vi "prep cmrcial shots report (SubVI).vi"(0 "reportType":enum32{"V50", "NIJ"}(ring), 1 "language":enum16{"Spanish", "Portuguese", "English"}(ring), 2 "shotsArr":T1 {"Frag Rod" format="%.1f"; "UncorrectedAvgVel_PB" format="%.1f"; "UncorrectedRed_PB" format="%.1f"; "strikeVel_PB" format="%.1f"; "velLoss_PB" format="%.1f"; "avgVel_PB" format="%.1f"; "Redundant_Velocity" format="%.1f"; "Energy Loss (J)" format="%.3e"; "Projectile Mass" min=0 step=1 format="%.4f"; "Corrected residual" format="%.2f"; "Uncorrected Residual" format="%.1f"; "Corrected Impact" format="%.2f"; "Uncorrected Impact" format="%.1f"; "Shot Angle" max=90 step=1; "SHOT STATUS" items=["Partial", "Complete"]; "IMPACT VELOCITY" min=0 max=10000 step=0.1 format="%.1f"; "Barrel Temperature" format="%.1f"; "Powder Loading" format="%.4f"; "RESIDUAL  VELOCITY" min=0 max=10000 step=0.1 format="%.1f"}) -> (3 "Custom Template":path, 4 "shotArrayOUT":string[][](array[string]))   [LabVIEW 2015]
uses:
  shotsArr.ctl
  Shot Record.ctl
panel:
  # "Corrected"
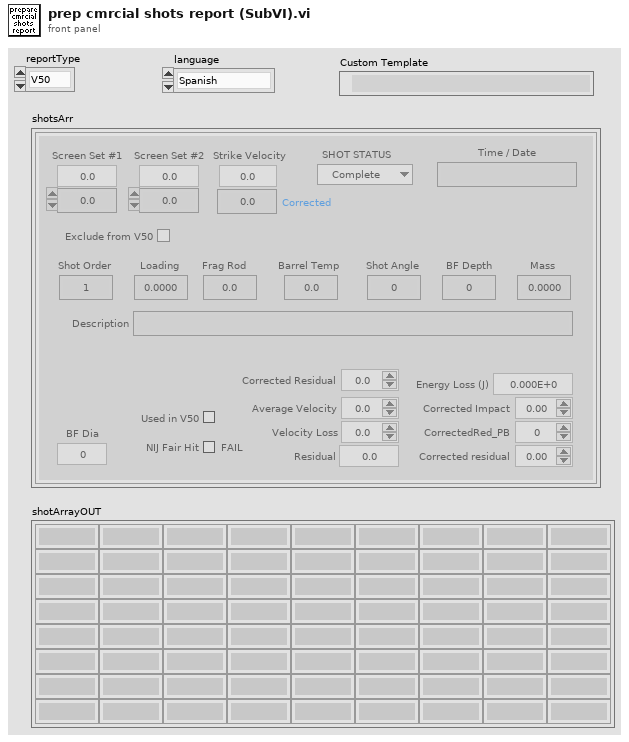
[diagram p1: front panel]
types:
  T1 = typedef "shotsArr.ctl" = T2[]
  T2 = typedef "Shot Record.ctl" = cluster{"Uncorrected Impact":sgl, "Uncorrected Residual":sgl, "avgVel_PB":sgl, "IMPACT VELOCITY":sgl, "RESIDUAL  VELOCITY ":sgl, "Shot Description":string, "Powder Loading ":sgl, "Barrel Temperature":sgl, "TIME / DATE":string, "shot order":i32, "SHOT STATUS":u16, "Shot Angle":u16, "Corrected Impact":sgl, "Corrected residual":sgl, "Projectile Mass":sgl, "usedv50":bool, "Energy Loss (J)":sgl, "BackFace\nDepth":sgl, "BackFace\nDiameter":sgl, "Redundant_Velocity":sgl, "velLoss_PB":sgl, "strikeVel_PB":sgl, "UncorrectedRed_PB":sgl, "CorrectedRed_PB":sgl, "UncorrectedAvgVel_PB":sgl, "V50userExcl":bool, "Frag Rod":sgl, "fairHit":bool}
  T3 = cluster{"[0]":string, "[1]":string, "[2]":string, "[3]":string, "[4]":string, "[5]":string, "[6]":string, "[7]":string, "[8]":string}[]
  T4 = cluster{"[0]":string, "[1]":string, "[2]":string, "[3]":string, "[4]":string, "[5]":string, "[6]":string, "[7]":string, "[8]":string}
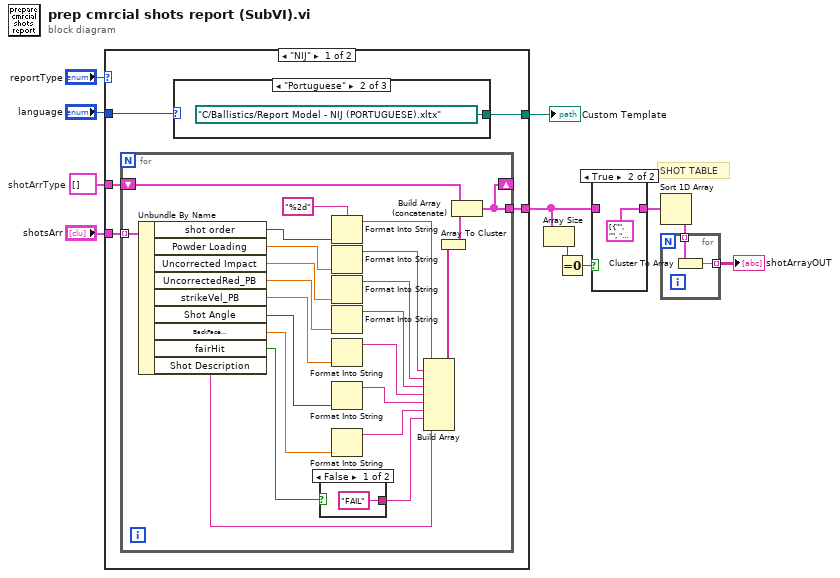
[diagram p0: block diagram]
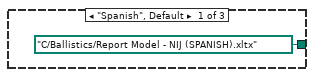
[diagram p2: hidden frame]
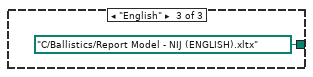
[diagram p3: hidden frame]
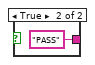
[diagram p4: hidden frame]
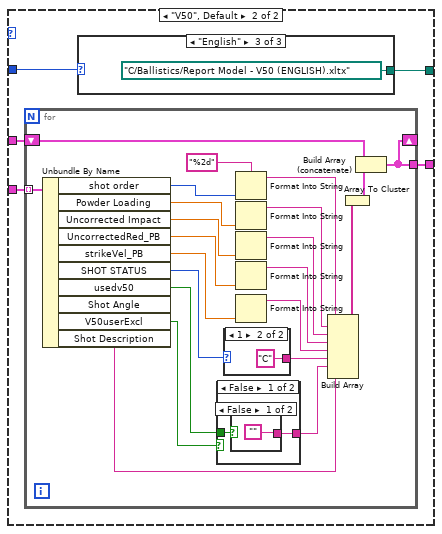
[diagram p5: hidden frame]
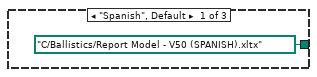
[diagram p6: hidden frame]
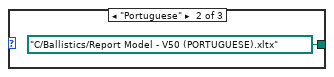
[diagram p7: hidden frame]
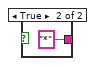
[diagram p8: hidden frame]
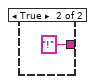
[diagram p9: hidden frame]
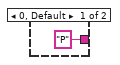
[diagram p10: hidden frame]
diagram:
  w1 = T3 []  # shotArrType
  # "SHOT TABLE"
  n1 = case shown="\"NIJ\"" "reportType" {
    tunnel: "shotsArr" -> [w16 w49]
    tunnel: [w15 w48] -> w4
    tunnel: w1 -> [w14 w47]
    tunnel: [w13 w46] -> w8
    tunnel: "language" -> [w12 w45]
    frame "NIJ" {
      n2 = for {
        tunnel: w16 -> [w42] mode=indexing
        shift-right: [w26] -> _
        shift-left: w14 -> [w28]
        tunnel: [w26] -> w15
        n3 = Unbundle By Name(w42) -> ("shot order"=w41:i32, "Powder Loading"=w40:sgl, "Uncorrected Impact"=w39:sgl, "UncorrectedRed_PB"=w38:sgl, "strikeVel_PB"=w37:sgl, "Shot Angle"=w23:u16, "BackFace\nDepth"=w24:sgl, "fairHit"=w21:bool, "Shot Description"=w22:string)
        n4 = case shown="False" w21 {
          tunnel: ["FAIL" "PASS"] -> w20
          frame False {
          }
          frame True {
          }
        }
        n5 = Format Into String(format string="%2d", w41) -> (resulting string=w31:string)  [unwired: 2 in, 1 out]
        n6 = Format Into String(w40) -> (resulting string=w32:string)  [unwired: 3 in, 1 out]
        n7 = Format Into String(w39) -> (resulting string=w33:string)  [unwired: 3 in, 1 out]
        n8 = Format Into String(w38) -> (resulting string=w34:string)  [unwired: 3 in, 1 out]
        n9 = Format Into String(w37) -> (resulting string=w35:string)  [unwired: 3 in, 1 out]
        n10 = Format Into String(w23) -> (resulting string=w36:string)  [unwired: 3 in, 1 out]
        n11 = Format Into String(w24) -> (resulting string=w30:string)  [unwired: 3 in, 1 out]
        n12 = Build Array(w31, w32, w33, w34, w35, w36, w30, w20, w22) -> (w27:string[])
        n13 = Array To Cluster(array=w27) -> (cluster=w29:T4)
        n14 = Build Array (concatenate)(w28, w29) -> (w26:T3)
      }
      n15 = case shown="\"Portuguese\"" w12 {
        tunnel: [path "C:/Ballistics/Report Model - NIJ (SPANISH).xltx" ("Custom Template") path "C:/Ballistics/Report Model - NIJ (PORTUGUESE).xltx" ("Custom Template") path "C:/Ballistics/Report Model - NIJ (ENGLISH).xltx" ("Custom Template")] -> w13
        frame "Spanish", Default {
        }
        frame "Portuguese" {
        }
        frame "English" {
        }
      }
    }
    frame "V50", Default {
      n16 = for {
        tunnel: w49 -> [w74] mode=indexing
        shift-right: [w56] -> _
        shift-left: w47 -> [w58]
        tunnel: [w56] -> w48
        n17 = Unbundle By Name(w74) -> ("shot order"=w73:i32, "Powder Loading"=w72:sgl, "Uncorrected Impact"=w71:sgl, "UncorrectedRed_PB"=w70:sgl, "strikeVel_PB"=w69:sgl, "SHOT STATUS"=w61:u16, "usedv50"=w68:bool, "V50userExcl"=w53:bool, "Shot Description"=w54:string)  [unwired: 1 out]
        n18 = case shown="False" w53 {
          tunnel: w68 -> [w76 _]
          tunnel: [w75 "!"] -> w67
          frame False {
            n19 = case shown="False" w76 {
              tunnel: ["" ("Empty String Constant") "*"] -> w75
              frame False {
              }
              frame True {
              }
            }
          }
          frame True {
          }
        }
        n20 = case shown="1" w61 {
          tunnel: ["P" "C"] -> w60
          frame 0, Default {
          }
          frame 1 {
          }
        }
        n21 = Format Into String(format string="%2d", w73) -> (resulting string=w62:string)  [unwired: 2 in, 1 out]
        n22 = Format Into String(w72) -> (resulting string=w63:string)  [unwired: 3 in, 1 out]
        n23 = Format Into String(w71) -> (resulting string=w64:string)  [unwired: 3 in, 1 out]
        n24 = Format Into String(w70) -> (resulting string=w65:string)  [unwired: 3 in, 1 out]
        n25 = Format Into String(w69) -> (resulting string=w66:string)  [unwired: 3 in, 1 out]
        n26 = Build Array(w62, w63, w64, w65, w66, w60, w67, w54) -> (w57:string[])
        n27 = Array To Cluster(array=w57) -> (cluster=w59:T4)
        n28 = Build Array (concatenate)(w58, w59) -> (w56:T3)
      }
      n29 = case shown="\"English\"" w45 {
        tunnel: [path "C:/Ballistics/Report Model - V50 (SPANISH).xltx" ("Custom Template") path "C:/Ballistics/Report Model - V50 (PORTUGUESE).xltx" ("Custom Template") path "C:/Ballistics/Report Model - V50 (ENGLISH).xltx" ("Custom Template")] -> w46
        frame "Spanish", Default {
        }
        frame "Portuguese" {
        }
        frame "English" {
        }
      }
    }
  }
  "Custom Template" <- w8
  n30 = Array Size(array=w4) -> (size(s)=w2:i32)
  n31 = Equal To 0?(x=w2) -> (x = 0?=w6:bool)
  n32 = case shown="True" w6 {
    tunnel: [w82 T3 [{"[0]"="", "[1]"="", "[2]"="", "[3]"="", "[4]"="", "[5]"="", "[6]"="", "[7]"="", "[8]"=""}]] -> w5
    tunnel: w4 -> [w82 _]
    frame False {
    }
    frame True {
    }
  }
  n33 = Sort 1D Array(array=w5) -> (sorted array=w3:T3)
  n34 = for {
    tunnel: w3 -> [w85] mode=indexing
    tunnel: [w84] -> w7 mode=indexing
    n35 = Cluster To Array(cluster=w85) -> (array=w84:string[])
  }
  "shotArrayOUT" <- w7
